vi "SENS_CORR_EXT_PORT_LDC.vi"(0 "VISA IN":refnum<visa-resource-name>, 1 "Port":i32, 2 "Loss(dB)":i32, 5 "error in":errorcluster, 7 "Channel":i32) -> (14 "VISA Out":refnum<visa-resource-name>, 19 "error out":errorcluster)   [LabVIEW 2018, in "PNA-X.lvlib"]
doc: "SENSe<cnum>:CORRection:EXTension:PORT<pnum>:LDC <value> \n(Read-Write) Sets and returns the Port Loss at DC value for the specified port number. \nLearn about Loss Compensation values. \nNote: This command affects ALL measurements on the specified channel. \nParameters \n<cnum> Any existing channel number. If unspecified, value is set to 1 \n<pnum> Port number to receive Loss value. If unspecified, value is set to 1. \n<value> Loss in dB. Choose a value between -90 and 90 \nExamples SENS:CORR:EXT:PORT:LDC 1.5 \nsense2:correction:extension:port2:ldc .1 \nQuery Syntax SENSe<cnum>:CORRection:EXTension:PORT<pnum>:LDC? \n1705\n\nReturn Type Numeric \nDefault 0"
uses:
  PNA-X.lvlib
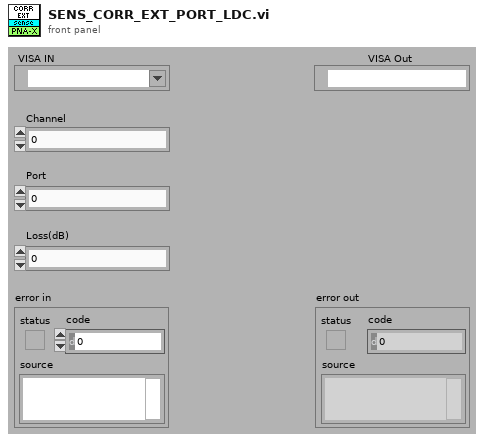
[diagram p1: front panel]
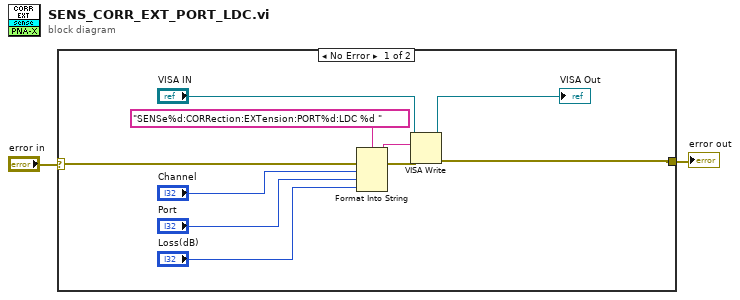
[diagram p0: block diagram]
diagram:
  n1 = case shown="No Error" "error in" {
    selector: "error in" -> [w12 w13]
    tunnel: [w7 w13] -> w1
    frame No Error {
      n2 = Format Into String(format string="SENSe%d:CORRection:EXTension:PORT%d:LDC %d " ("Cmdline"), error in=w12, "Channel", "Port", "Loss(dB)") -> (resulting string=w10:string, error out=w11:errorcluster)  [unwired: 1 in]
      n3 = VISA Write(VISA resource name="VISA IN", write buffer=w10, error in (no error)=w11) -> (VISA resource name out=→"VISA Out":refnum<visa-resource-name>, error out=w7:errorcluster)  [unwired: 1 out]
    }
    frame Error {
    }
  }
  "error out" <- w1
